vi "Dialog Properties.vi"(8 "error in (no error)":errorcluster, 9 "Boolean":bool, 11 "reference":refnum<vi>) -> (0 "error out":errorcluster, 3 "reference out":refnum<vi>)   [LabVIEW 2018]
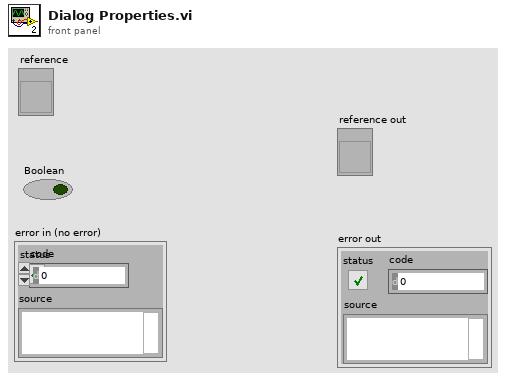
[diagram p1: front panel]
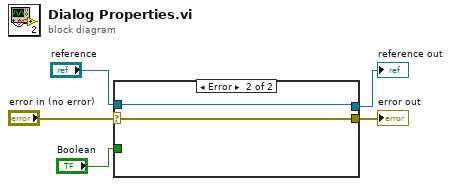
[diagram p0: block diagram]
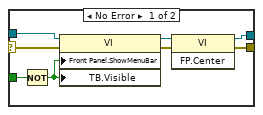
[diagram p2: hidden frame]
diagram:
  n1 = case shown="Error" "error in (no error)" {
    selector: "error in (no error)" -> [w12 w14]
    tunnel: "reference" -> [w13 w15]
    tunnel: [w9 w14] -> w3
    tunnel: [w8 w15] -> w2
    tunnel: "Boolean" -> [w7 _]
    frame No Error {
      n2 = Not(x=w7) -> (.not. x?=w6:bool)
      n3 = property class="VI"(reference=w13, error in=w12, "Front Panel.ShowMenuBar"=w6, "TB.Visible"=w6) -> (reference out=w11:refnum<vi>, error out=w10:errorcluster)
      n4 = invoke class="VI" method="FP.Center"(reference=w11, error in=w10) -> (reference out=w8:refnum<vi>, error out=w9:errorcluster)  [unwired: 1 in, 1 out]
    }
    frame Error {
    }
  }
  "reference out" <- w2
  "error out" <- w3
